vi "DAQmx Create Channel (TEDS-AI-Current-Basic).vi"(0 "task in":refnum<k21>, 1 "maximum value":dbl=0.01 format="%0.5f", 2 "minimum value":dbl=-0.01 format="%0.5f", 3 "input terminal configuration":i32(ring)=-1 items=["default"=-1, "RSE"=10083, "NRSE"=10078, "Differential"=10106, "Pseudodifferential"=12529], 5 "physical channels":tag, 7 "name to assign":string, 8 "external shunt resistor value":dbl=249.0 format="%0.2f", 9 "units":i32(ring)=12516 items=["From TEDS"=12516, "From Custom Scale"=10065], 11 "error in":errorcluster, 12 "custom scale name":tag, 14 "shunt resistor location":i32(ring)=-1 items=["default"=-1, "Internal"=10200, "External"=10167]) -> (4 "task out":refnum<k21>, 15 "error out":errorcluster)   [LabVIEW 2013]
doc: "Creates channel(s) to measure current. You must configure the physical channel(s) with TEDS information to use this VI."
uses:
  <resource>/objmgr/daqmx.rc
panel:
  # "input limits"
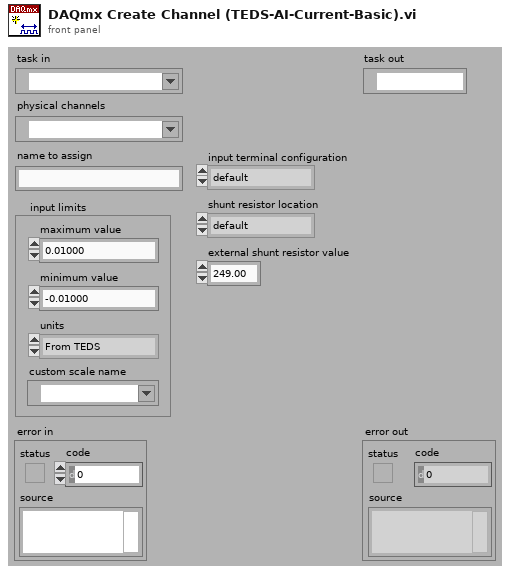
[diagram p1: front panel]
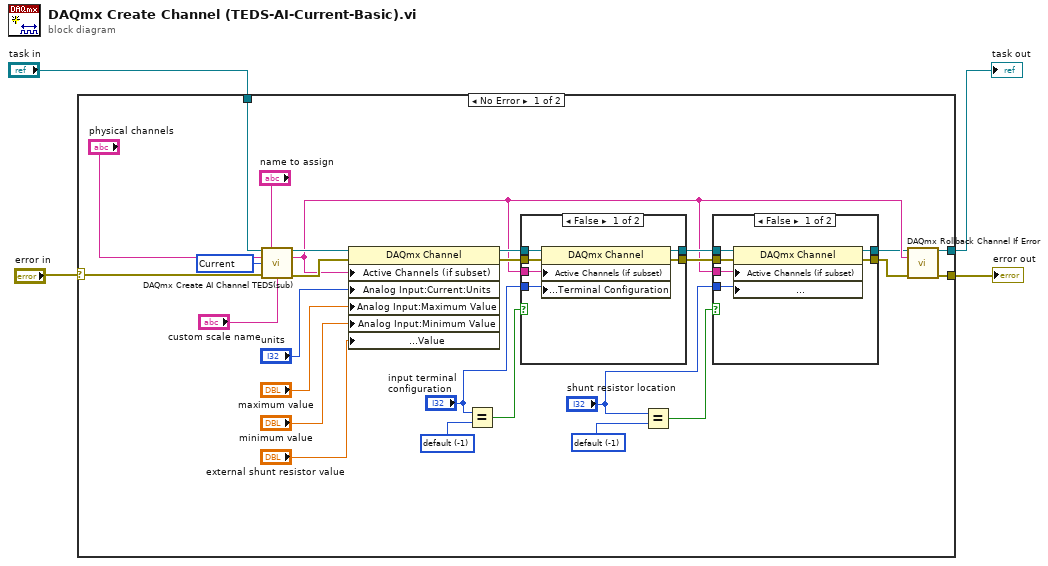
[diagram p0: block diagram]
diagram:
  n1 = case shown="No Error" "error in" {
    selector: "error in" -> [w30 w49]
    tunnel: [w14 w49] -> w4
    tunnel: [w15 w48] -> w3
    tunnel: "task in" -> [w29 w48]
    frame No Error {
      w12 = -1 items=["default"=-1, "Internal"=10200, "External"=10167] ("shunt resistor location")
      w13 = 10134 items=["Voltage"=10322, "Current"=10134, "More:Voltage:Custom with Excitation"=10323, "More:Current:Custom with Excitation"=10136, "Frequency"=10181, "Period"=10257, "Resistance"=10278, "Temperature:Thermocouple"=10303, "Temperature:Thermistor"=10302, "Temperature:RTD"=10301, "Temperature:Built-in Sensor"=10311, "Strain Gage"=10300, "LVDT"=10352, "RVDT"=10353, "Accelerometer:Voltage Input"=10355, "Accelerometer:Current Input"=10356, "Sound Pressure:Microphone"=10354, "TEDS"=12531] ("measurement type")
      w18 = -1 items=["default"=-1, "differential"=10106, "RSE"=10083, "NRSE"=10078] ("input terminal configuration")
      n2 = call "DAQmx Create AI Channel TEDS(sub).vi"("task in"=w29, "virtual channel name"="name to assign", "physical channel name"="physical channels", "measurement type"=w13, "error in"=w30, "custom scale"="custom scale name") -> ("task out"=w16:refnum<k21>, "channel names"=w8:string, "error out"=w28:errorcluster)  [unwired: 7 out]
      n3 = property class="DAQmx Channel"(reference=w16, error in=w28, "Active Channels (if subset)"=w8, "Analog Input:Current:Units"="units", "Analog Input:Maximum Value"="maximum value", "Analog Input:Minimum Value"="minimum value", "Analog Input:General Properties:Signal Conditioning:Current Shunt Resistor:Value"="external shunt resistor value") -> (reference out=w23:refnum<k21>, error out=w22:errorcluster)
      n4 = Equal?(x="input terminal configuration", y=w18) -> (x = y?=w24:bool)
      n5 = case shown="False" w24 {
        tunnel: "input terminal configuration" -> [w42 _]
        tunnel: w23 -> [w40 w47]
        tunnel: [w45 w47] -> w10
        tunnel: w22 -> [w44 w46]
        tunnel: [w43 w46] -> w9
        tunnel: w8 -> [w41 _]
        frame False {
          n6 = property class="DAQmx Channel"(reference=w40, error in=w44, "Active Channels (if subset)"=w41, "Analog Input:General Properties:Input Configuration:Terminal Configuration"=w42) -> (reference out=w45:refnum<k21>, error out=w43:errorcluster)
        }
        frame True {
        }
      }
      n7 = Equal?(x="shunt resistor location", y=w12) -> (x = y?=w11:bool)
      n8 = case shown="False" w11 {
        tunnel: "shunt resistor location" -> [w34 _]
        tunnel: w10 -> [w32 w39]
        tunnel: [w37 w39] -> w6
        tunnel: w9 -> [w36 w38]
        tunnel: [w35 w38] -> w5
        tunnel: w8 -> [w33 _]
        frame False {
          n9 = property class="DAQmx Channel"(reference=w32, error in=w36, "Active Channels (if subset)"=w33, "Analog Input:General Properties:Signal Conditioning:Current Shunt Resistor:Location"=w34) -> (reference out=w37:refnum<k21>, error out=w35:errorcluster)
        }
        frame True {
        }
      }
      n10 = call "DAQmx Rollback Channel If Error.vi"("task in"=w6, "channel names"=w8, "error in"=w5) -> ("task out"=w15:refnum<k21>, "error out"=w14:errorcluster)  [unwired: 11 out]
    }
    frame Error {
    }
  }
  "error out" <- w4
  "task out" <- w3
